vi "MQTT Chat Launcher.vi"() -> ()   [LabVIEW 2020, in "Simple Chat.lvlib"]
uses:
  Simple Chat.lvlib
  Simple Chat/Simple Chat.lvclass
  C:/Program Files (x86)/National Instruments/LabVIEW 2020/vi.lib/ActorFramework/Actor/Actor.lvclass
  <vilib>/LabVIEW Open Source Project/MQTT Control Packets/Control Packets/CONNECT/ConnectFlags -- cluster.ctl
  <vilib>/LabVIEW Open Source Project/MQTT Client/Client class/Client.lvclass/Client.ctl
  <vilib>/LabVIEW Open Source Project/MQTT Broker/Server class/Server.lvclass/Server.ctl
  <vilib>/LabVIEW Open Source Project/MQTT Control Packets/Control Packets/ControlPacket/ControlPacket.lvclass/ControlPacket.ctl
  <vilib>/ActorFramework/Message Enqueuer/Message Enqueuer.lvclass/Message Enqueuer.ctl
  <vilib>/ActorFramework/Message Enqueuer/Enqueue.vi
  <vilib>/LabVIEW Open Source Project/MQTT TCP Connection/MQTT_TCP/Connection/TCPConnection.lvclass
  C:/Program Files (x86)/National Instruments/LabVIEW 2020/vi.lib/LabVIEW Open Source Project/MQTT Connection/MQTT_Connection/Connection/Connection.lvclass
  <vilib>/LabVIEW Open Source Project/MQTT Client/Client class/Client.lvclass
  C:/Program Files (x86)/National Instruments/LabVIEW 2020/vi.lib/LabVIEW Open Source Project/MQTT Connection/MQTT_Base/Base Class/MQTT_Base.lvclass
  <vilib>/LabVIEW Open Source Project/MQTT Broker/Server class/Server.lvclass
  AF MQTT Channel/AF MQTT Message Channel/AF MQTT Message Channel.lvclass
  C:/Users/Simon/Documents/GitHub/LV-Actor-Pub-Sub/Source/Actor Pub Sub Channels/Pub Sub Message Channel/Pub Sub Message Channel.lvclass
  <vilib>/LabVIEW Open Source Project/MQTT Control Packets/Control Packets/PUBLISH/PUBLISH.lvclass
  C:/Program Files (x86)/National Instruments/LabVIEW 2020/vi.lib/LabVIEW Open Source Project/MQTT Control Packets/Control Packets/ControlPacket/ControlPacket.lvclass
  <vilib>/ActorFramework/Stop Msg/Stop Msg.lvclass
  C:/Program Files (x86)/National Instruments/LabVIEW 2020/vi.lib/ActorFramework/Message/Message.lvclass
  Actor Pub Sub Channels/Helpers/Get Topic Enqueuer.vi
  <vilib>/ActorFramework/Message Priority Queue/Priority Enqueue.vi
  <vilib>/LabVIEW Open Source Project/MQTT Connection/MQTT_Base/Base Class/MQTT_Base.lvclass
  <vilib>/ActorFramework/Actor/Actor.lvclass
  Actor Pub Sub Channels/Actor Pub Sub Channels.lvlib
  <vilib>/LabVIEW Open Source Project/MQTT Control Packets/Control Packets/CONNECT/CONNECT.lvclass
  C:/Users/Simon/Documents/GitHub/LV-Actor-Pub-Sub/Source/AF MQTT Channel/AF MQTT Message Channel/AF MQTT Message Channel.lvclass
  C:/Program Files (x86)/National Instruments/LabVIEW 2020/vi.lib/LabVIEW Open Source Project/MQTT TCP Connection/MQTT_TCP/Connection/TCPConnection.lvclass
  <vilib>/LabVIEW Open Source Project/MQTT Control Packets/Control Packets/ControlPacket/ControlPacket.lvclass
  C:/Program Files (x86)/National Instruments/LabVIEW 2020/vi.lib/LabVIEW Open Source Project/MQTT Broker/Server class/Server.lvclass
  C:/Program Files (x86)/National Instruments/LabVIEW 2020/vi.lib/LabVIEW Open Source Project/MQTT Client/Client class/Client.lvclass
  C:/Users/Simon/Documents/GitHub/LV-Actor-Pub-Sub/Source/Simple Chat/Simple Chat/Simple Chat.lvclass
  C:/Users/Simon/Documents/GitHub/LV-Actor-Pub-Sub/Source/Actor Pub Sub Channels/PubSub Status Reciever Interface/PubSub Status Reciever Interface.lvclass
  C:/Users/Simon/Documents/GitHub/LV-Actor-Pub-Sub/Source/Simple Chat/Message Reciever Interface/Message Reciever Interface.lvclass
  C:/Program Files (x86)/National Instruments/LabVIEW 2020/vi.lib/LabVIEW Open Source Project/MQTT Control Packets/Control Packets/PUBLISH/PUBLISH.lvclass
panel:
  out "String":string
  in  "stop":bool
  in  "Boolean":bool
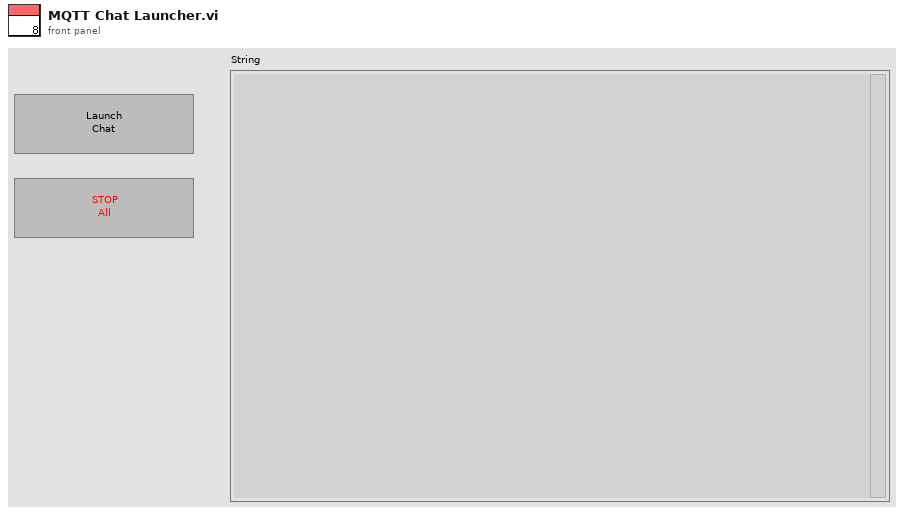
[diagram p1: front panel]
types:
  T1 = typedef "MQTT_Control_Packets.lvlib/CONNECT.lvclass/ConnectFlags -- cluster.ctl" = cluster{"Reserved":bool, "Clean Session":bool, "Will Flag":bool, "Will QoS 1":bool, "Will QoS 2":bool, "Will Retain":bool, "Password Flag":bool, "User Name Flag":bool}
  T2 = typedef "MQTT Server.lvlib/Server.lvclass/Public Events -- cluster.ctl" = cluster{"NbConnections":refnum<user-event>}
  T3 = typedef "MQTT Client.lvlib/Client.lvclass/Public Events -- cluster.ctl" = cluster{"Connection Status":refnum<user-event>, "Connected":refnum<user-event>, "Application Message":refnum<user-event>}
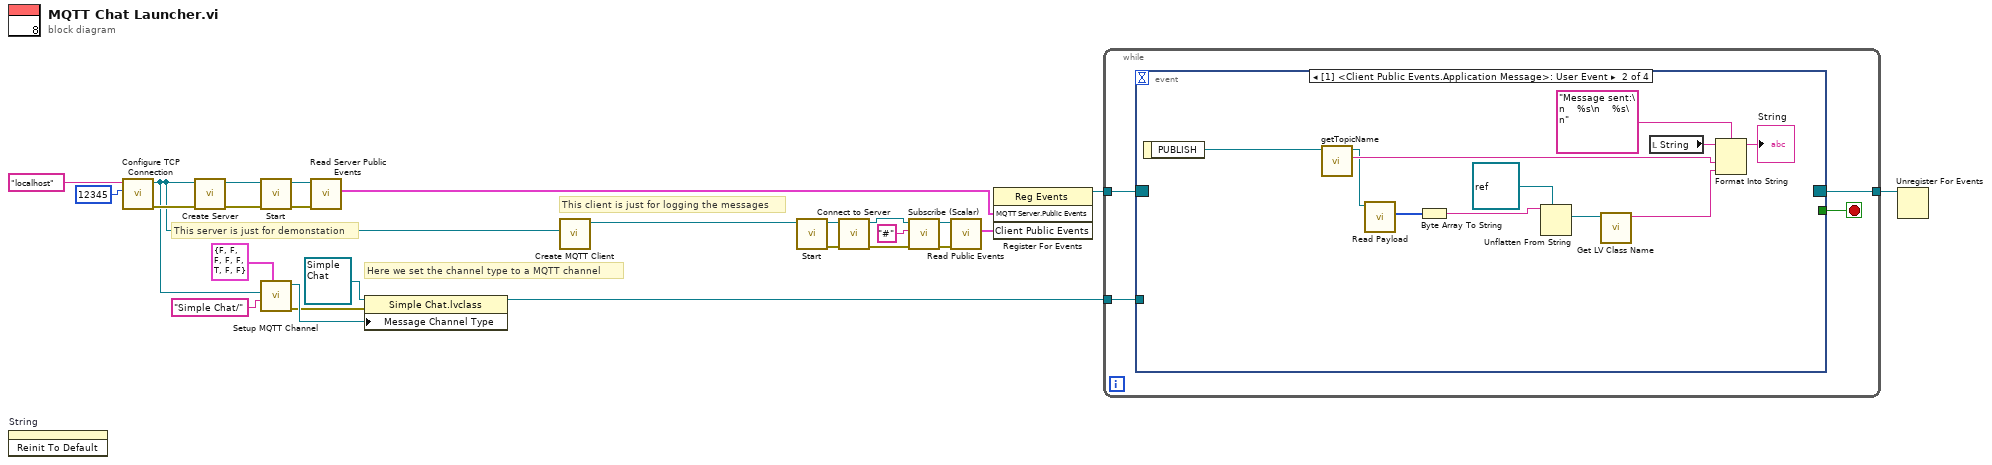
[diagram p0: block diagram]
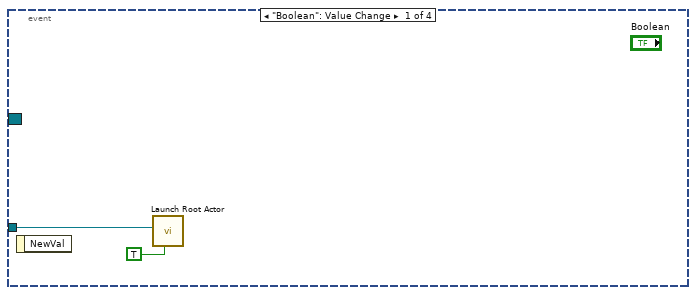
[diagram p2: hidden frame]
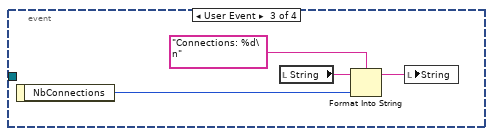
[diagram p3: hidden frame]
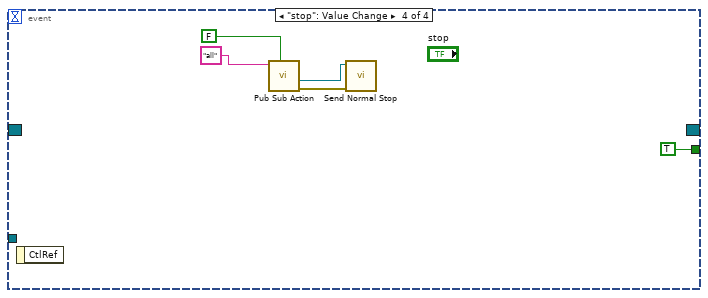
[diagram p4: hidden frame]
diagram:
  # "Here we set the channel type to a MQTT channel"
  # "This server is just for demonstation"
  # "This client is just for logging the messages"
  n1 = invoke on="String" class="Str" method="Reinit To Default"() -> ()  [unwired: 3 in, 3 out]
  n2 = call <vilib>:"Configure TCP Connection.vi"("remote port (80)"=u16 12345, "address (localhost)"="localhost") -> ("error out"=w24:errorcluster, "TCPConnection"=w10:refnum<class "TCPConnection.lvclass">)  [unwired: 8 in]
  n3 = call <vilib>:"Create Server.vi"("error in (no error)"=w24, "Connection Configuration"=w10) -> ("error out"=w22:errorcluster, "Server"=w23:refnum<class "Server.lvclass">)  [unwired: 8 in]
  n4 = call <vilib>:"Start.vi"("error in (no error)"=w22, "MQTT_Base in"=w23) -> ("error out"=w16:errorcluster, "MQTT_Base out"=w17:refnum<class "Server.lvclass">)  [unwired: 7 in, 1 out]
  n5 = call "Setup MQTT Channel.vi"("Connect Flags"=T1 {"Reserved"=FALSE, "Clean Session"=FALSE, "Will Flag"=FALSE, "Will QoS 1"=FALSE, "Will QoS 2"=FALSE, "Will Retain"=TRUE, "Password Flag"=FALSE, "User Name Flag"=FALSE}, "Topic Prefix"="Simple Chat/", "Connection Configuration"=w10) -> ("error out"=w18:errorcluster, "AF MQTT Message Channel out"=w19:refnum<class "AF MQTT Message Channel.lvclass">)  [unwired: 7 in]
  n6 = call <vilib>:"Read Server Public Events.vi"("error in (no error)"=w16, "Server in"=w17) -> ("MQTT Server.Public Events"=w13:T2)  [unwired: 7 in, 2 out]
  n7 = property class="Simple Chat.lvclass"(reference=refnum<class "Simple Chat.lvclass"> refnum ("Simple Chat.lvlib:Simple Chat.lvclass"), error in=w18, "Message Channel Type"=w19) -> (reference out=w20:refnum<class "Simple Chat.lvclass">)  [unwired: 1 out]
  n8 = call <vilib>:"Create MQTT Client.vi"("Connection Configuration"=w10) -> ("Client out"=w9:refnum<class "Client.lvclass">)  [unwired: 9 in, 1 out]
  n9 = call <vilib>:"Start.vi"("MQTT_Base in"=w9) -> ("error out"=w7:errorcluster, "MQTT_Base out"=w8:refnum<class "Client.lvclass">)  [unwired: 8 in, 1 out]
  n10 = call <vilib>:"Connect to Server.vi"("error in (no error)"=w7, "Client in"=w8) -> ("error out"=w5:errorcluster, "Client out"=w6:refnum<class "Client.lvclass">)  [unwired: 6 in, 2 out]
  n11 = call <vilib>:"Subscribe (Scalar).vi"("error in (no error)"=w5, "Topic Filter"="#", "Client in"=w6) -> ("error out"=w2:errorcluster, "Client out"=w3:refnum<class "Client.lvclass">)  [unwired: 6 in, 1 out]
  n12 = call <vilib>:"Read Public Events.vi"("error in (no error)"=w2, "Client in"=w3) -> ("Client Public Events"=w1:T3)  [unwired: 7 in, 2 out]
  n13 = register-events(w13, w1) -> (reference out=w15:refnum<event-registration>)  [unwired: 2 in, 1 out]
  n14 = while {
    tunnel: w20 -> [w30]
    tunnel: w15 -> [w29]
    tunnel: [w28] -> w14
    stop <- w27 stop-if-true
    n15 = event shown="[1] <Client Public Events.Application Message>: User Event" {
      selector: w29 -> [_ _ _ _]
      dyn-events: [_ _ _ _] -> w28
      timeout: _ -> [_ _ _ _]
      tunnel: w30 -> [w31 _ _ _]
      tunnel: [_ _ _ TRUE] -> w27
      event "Boolean": Value Change {
        n16 = event-data() -> ()  [unwired: 1 in, 1 out]
        n17 = call <vilib>:"Launch Root Actor.vi"("Open Actor Core front panel? (F)"=TRUE, "Actor"=w31) -> ()  [unwired: 8 in, 2 out]
      }
      event User Event {
        n18 = event-data() -> ("PUBLISH"=w43:refnum<class "PUBLISH.lvclass">)  [unwired: 1 in]
        n19 = call <vilib>:"getTopicName.vi"("PUBLISH in"=w43) -> ("Topic"=w40:string, "PUBLISH out"=w38:refnum<class "PUBLISH.lvclass">)  [unwired: 8 in, 1 out]
        n20 = call <vilib>:"Read Payload.vi"("ControlPacket in"=w38) -> ("Payload"=w37:u8[])  [unwired: 9 in, 1 out]
        n21 = Byte Array To String(unsigned byte array=w37) -> (string=w36:string)
        n22 = Unflatten From String(type=refnum<class> refnum ("LabVIEW Object"), binary string=w36) -> (value=w34:refnum<class>)  [unwired: 3 in, 2 out]
        n23 = call <vilib>:"Get LV Class Name.vi"("object"=w34) -> ("class name"=w33:string)  [unwired: 9 in, 1 out]
        n24 = local read "String"() -> (w42:string)
        n25 = Format Into String(format string="Message sent:\n    %s\n    %s\n", initial string=w42, w40, w33) -> (resulting string=→"String":string)  [unwired: 1 in, 1 out]
      }
      event User Event {
        n26 = event-data() -> ("NbConnections"=w45:u32)  [unwired: 1 in]
        n27 = local read "String"() -> (w47:string)
        n28 = Format Into String(format string="Connections: %d\n", initial string=w47, w45) -> (resulting string=w44:string)  [unwired: 1 in, 1 out]
        n29 = local write "String"(w44) -> ()
      }
      event "stop": Value Change {
        n30 = event-data() -> ()  [unwired: 1 in, 1 out]
        n31 = call-poly "Pub Sub Action.vi"("Create if not exist? (T)"=FALSE, "Topic"="all") -> ("error out"=w50:errorcluster, "Topic Enqueuer"=w51:refnum<class "Message Enqueuer.lvclass">)  [unwired: 6 in, 2 out]
        n32 = call <vilib>:"Send Normal Stop.vi"("error in (no error)"=w50, "Message Enqueuer"=w51) -> ()  [unwired: 9 in, 1 out]
      }
    }
  }
  n33 = Unregister For Events(event registration refnum=w14) -> ()  [unwired: 1 in, 1 out]
